vi "SPI Init.vi"(9 "pConfig":T1, 10 "SPIIndex":i32, 11 "DevHandle":i32) -> (1 "pConfig out":T1, 3 "function return":i32)   [LabVIEW 2010, in "usb2spi.lvlib"]
doc: "int WINAPI SPI_Init(int DevHandle,int SPIIndex, PSPI_CONFIG pConfig);"
uses:
  usb2spi.lvlib
  USB2XXX/trunk/USB2XXX/USB2XXX/vs2019/Release/USB2XXX.dll
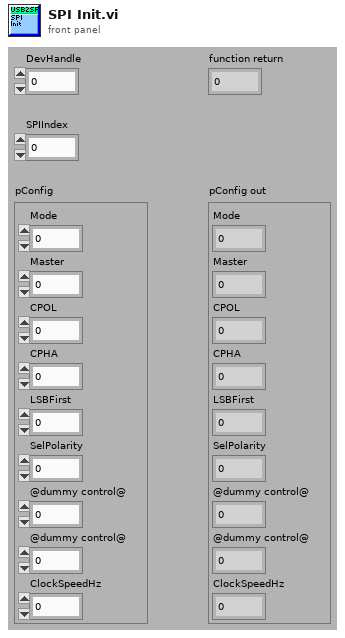
[diagram p1: front panel]
types:
  T1 = cluster{"Mode":i8, "Master":i8, "CPOL":i8, "CPHA":i8, "LSBFirst":i8, "SelPolarity":i8, "@dummy control@":i8, "@dummy control@":i8, "ClockSpeedHz":u32}
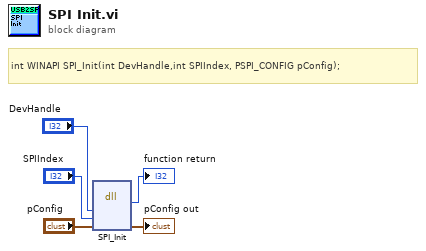
[diagram p0: block diagram]
diagram:
  # "int WINAPI SPI_Init(int DevHandle,int SPIIndex, PSPI_CONFIG pConfig);"
  n1 = dll-call lib="E:/Projects/USB2XXX/trunk/USB2XXX/USB2XXX/vs2019/Release/USB2XXX.*" fn="SPI_Init"("DevHandle"="DevHandle", "SPIIndex"="SPIIndex", "pConfig"="pConfig") -> (→"function return":i32, "pConfig"=→"pConfig out":T1)  [unwired: 5 in, 2 out]
